vi "Error Eater.vi"(2 "error in (no error)":errorcluster) -> ()   [LabVIEW 2012, in "Win8uiFramework.lvlib"]
uses:
  Win8uiFramework.lvlib
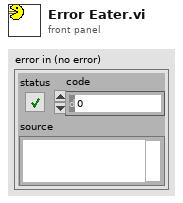
[diagram p1: front panel]
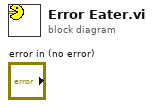
[diagram p0: block diagram]
diagram:
